vi "Configure Power Measurement Parameter Set.vi"(4 "Offset":dbl[](array[numeric]) format="%^.3e", 5 "Measurement Length":dbl[](array[numeric]) format="%^.3e", 6 "Step Length":dbl[](array[numeric]) format="%^.3e", 7 "Filter Type":u32[](array[numeric]), 8 "error in (no error)":errorcluster, 9 "Array Size (32)":i32=32, 10 "Instance (1)":i32=1, 11 "VISA resource name":refnum<visa-resource-name>) -> (0 "error out":errorcluster, 3 "VISA resource name out":refnum<visa-resource-name>)   [LabVIEW 2020, in "Rohde&Schwarz CMXP GPRF.lvlib"]
doc: "This VI sets is a combination of measurement control settings. The \"Parameter Set List\" contains 32 possibly different parameter sets which you may assign to the individual measurement steps in list mode.\n\nAttributes:\nRSCMXPGPRF_ATTR_POWER_MEASUREMENT_PARAMETER_SET_FILTER_TYPE_ALL\nRSCMXPGPRF_ATTR_POWER_MEASUREMENT_PARAMETER_SET_STEP_LENGTH_ALL\nRSCMXPGPRF_ATTR_POWER_MEASUREMENT_PARAMETER_SET_MEASUREMENT_LENGTH_ALL\nRSCMXPGPRF_ATTR_POWER_MEASUREMENT_PARAMETER_SET_OFFSET_ALL\n\nRemote-control commands:\nCONFigure:GPRF:MEAS<i>:POWer:PSET:FILTer:TYPE:ALL\nCONFigure:GPRF:MEAS<i>:POWer:PSET:SLENgth:ALL\nCONFigure:GPRF:MEAS<i>:POWer:PSET:MLENgth:ALL\nTRIGger:GPRF:MEAS<i>:POWer:PSET:OFFSet:ALL"
uses:
  <instrlib>/Rohde&Schwarz CMXP GPRF/Rohde&Schwarz CMXP GPRF.lvlib
  <instrlib>/Rohde&Schwarz CMXP GPRF/Private/rsidr_core.llb/rsidr_core.lvlib
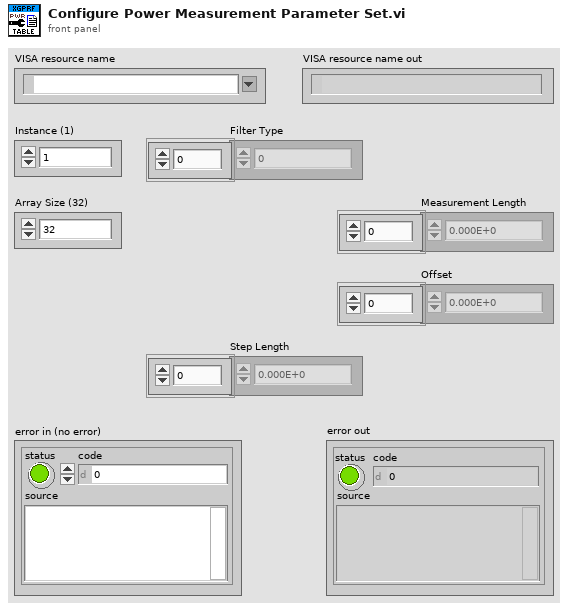
[diagram p1: front panel]
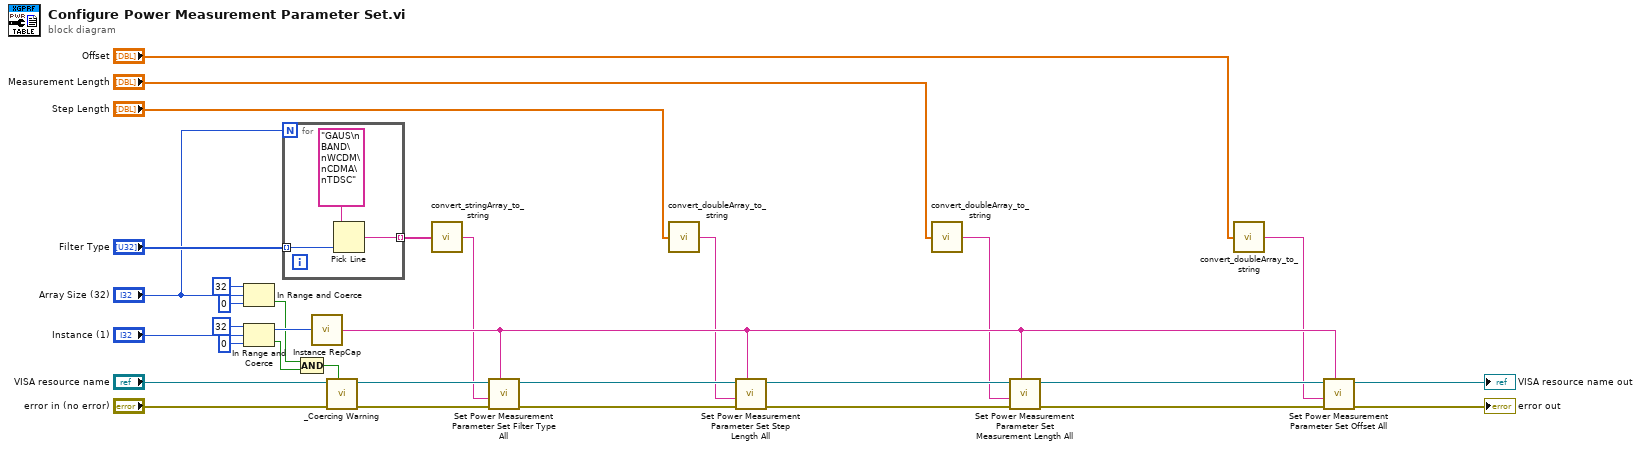
[diagram p0: block diagram]
diagram:
  n1 = In Range and Coerce(upper limit=32, x="Array Size (32)", lower limit=0) -> (In Range?=w5:bool)  [unwired: 1 out]
  n2 = In Range and Coerce(upper limit=32, x="Instance (1)", lower limit=0) -> (coerced(x)=w18:i32, In Range?=w6:bool)
  n3 = for {
    N: "Array Size (32)" -> [_]
    tunnel: "Filter Type" -> [w33] mode=indexing
    tunnel: [w34] -> w23 mode=indexing
    n4 = Pick Line(multi-line string="GAUS\n BAND\nWCDM\nCDMA\nTDSC", line index=w33) -> (output string=w34:string)  [unwired: 1 in]
  }
  n5 = Compound Arithmetic op=AND(w5, w6) -> (w28:bool)
  n6 = call <instrlib>:"Instance RepCap.vi"("Instance in"=w18) -> ("Instance out"=w7:string)
  n7 = call <instrlib>:"_Coercing Warning.vi"("In Range?"=w28, "error in (no error)"="error in (no error)", "VISA resource name"="VISA resource name") -> ("error out"=w17:errorcluster, "VISA resource name out"=w16:refnum<visa-resource-name>)  [unwired: 7 in]
  n8 = call <instrlib>:"convert_stringArray_to_string.vi"("string array in"=w23) -> ("string out"=w1:string)  [unwired: 4 in]
  n9 = call "Set Power Measurement Parameter Set Filter Type All"("Repeated Capabilities"=w7, "error in (no error)"=w17, "Power Measurement Parameter Set Filter Type All ()"=w1, "instrument handle"=w16) -> ("error out"=w15:errorcluster, "instrument handle out"=w14:refnum<visa-resource-name>)  [unwired: 6 in]
  n10 = call <instrlib>:"convert_doubleArray_to_string.vi"("double array in"="Step Length") -> ("string out"=w2:string)  [unwired: 4 in]
  n11 = call "Set Power Measurement Parameter Set Step Length All"("Repeated Capabilities"=w7, "error in (no error)"=w15, "Power Measurement Parameter Set Step Length All ()"=w2, "instrument handle"=w14) -> ("error out"=w13:errorcluster, "instrument handle out"=w12:refnum<visa-resource-name>)  [unwired: 6 in]
  n12 = call <instrlib>:"convert_doubleArray_to_string.vi"("double array in"="Measurement Length") -> ("string out"=w3:string)  [unwired: 4 in]
  n13 = call "Set Power Measurement Parameter Set Measurement Length All"("Repeated Capabilities"=w7, "error in (no error)"=w13, "Power Measurement Parameter Set Measurement Length All ()"=w3, "instrument handle"=w12) -> ("error out"=w11:errorcluster, "instrument handle out"=w10:refnum<visa-resource-name>)  [unwired: 6 in]
  n14 = call <instrlib>:"convert_doubleArray_to_string.vi"("double array in"="Offset") -> ("string out"=w4:string)  [unwired: 4 in]
  n15 = call "Set Power Measurement Parameter Set Offset All"("Repeated Capabilities"=w7, "error in (no error)"=w11, "Power Measurement Parameter Set Offset All ()"=w4, "instrument handle"=w10) -> ("error out"=→"error out":errorcluster, "instrument handle out"=→"VISA resource name out":refnum<visa-resource-name>)  [unwired: 6 in]
